vi "test Set and Get Options with GE Reflective Memory.vi"(8 "error in (no error)":errorcluster, 11 "TestCase in":refnum<class "Set and Get Config Options Test.lvclass">) -> (0 "error out":errorcluster, 3 "TestCase out":refnum<class "Set and Get Config Options Test.lvclass">)   [LabVIEW 2017, in "Set and Get Config Options Test.lvclass"]
uses:
  Set and Get Config Options Test.lvclass
  NationalInstruments.VeriStand.SystemDefinitionAPI
  <vilib>/addons/_JKI Toolkits/VI Tester/TestCase.llb/TestCase.lvclass
  niveristand-custom-device-testing-tools/VeriStandTestUtilities/VeriStandTestUtilities.lvlib
  C:/Program Files (x86)/National Instruments/LabVIEW 2017/vi.lib/addons/_JKI Toolkits/VI Tester/TestCase.llb/TestCase.lvclass
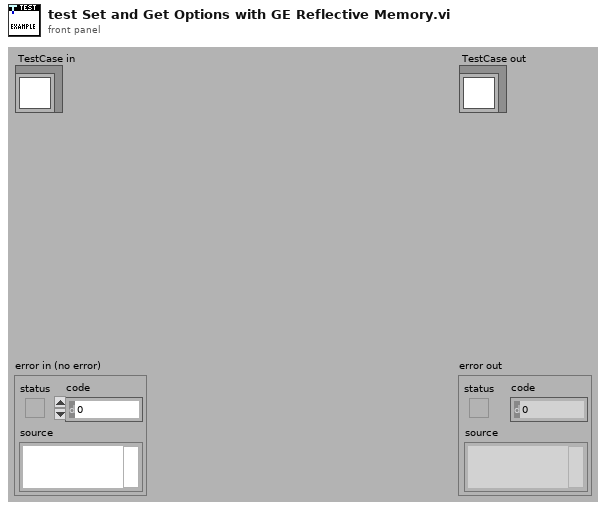
[diagram p1: front panel]
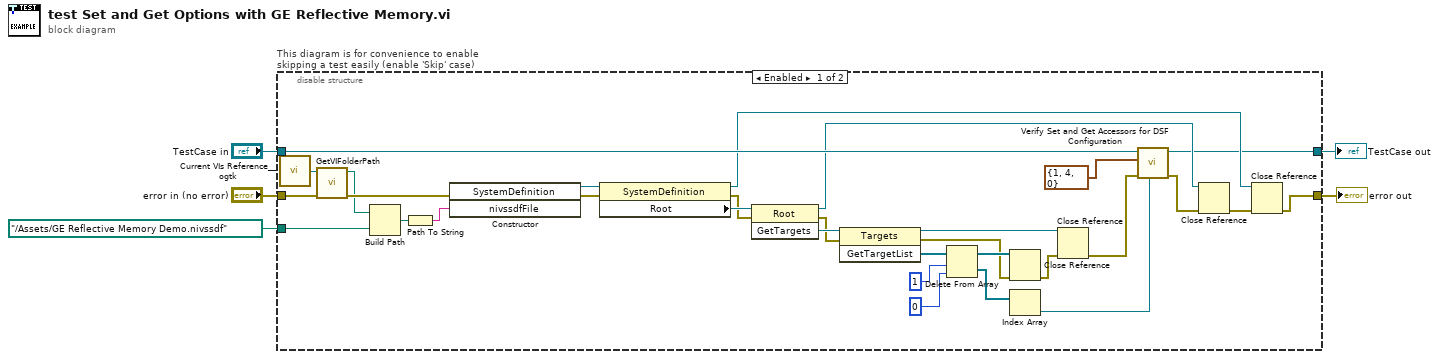
[diagram p0: block diagram]
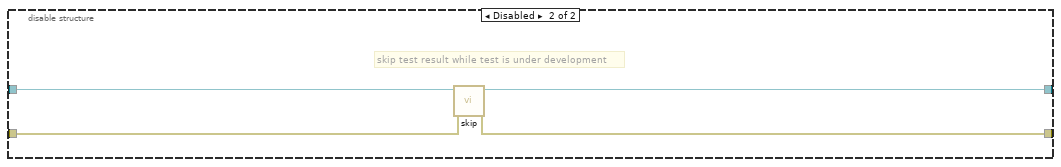
[diagram p2: hidden frame]
diagram:
  n1 = disable-structure "This diagram is for convenience to enable skipping a test easily (enable 'Skip' case)" shown="Enabled" {
    disable-tunnel: "TestCase in" -> [w36 w40]
    disable-tunnel: [w8 w38] -> w2
    disable-tunnel: [w10 w39] -> w4
    disable-tunnel: "error in (no error)" -> [w16 w37]
    disable-tunnel: path "../Assets/GE Reflective Memory Demo.nivssdf" ("Absolute or Relative Path") -> [w17 _]
    frame Enabled {
      n2 = call <userlib>:"Current VIs Reference__ogtk.vi"() -> ("Current VI's reference"=w19:refnum<vi>)  [unwired: 5 in]
      n3 = call "GetVIFolderPath.vi"("error in (no error)"=w16, "VI Reference in"=w19) -> ("error out"=w22:errorcluster, "VI Folder Path out"=w20:path)  [unwired: 8 in]
      n4 = Build Path(base path=w20, name or relative path=w17) -> (appended path=w21:path)
      n5 = Path To String(path=w21) -> (string=w24:string)
      n6 = constructor class="SystemDefinition" ("Constructor Node")(error in=w22, "nivssdfFile"=w24) -> (reference out=w25:refnum<k24>, error out=w23:errorcluster)  [unwired: 2 in, 2 out]
      n7 = property on="Property Node" class="SystemDefinition"(reference=w25, error in=w23) -> (reference out=w13:refnum<k24>, error out=w26:errorcluster, "Root"=w27:refnum<k24>)
      n8 = invoke on="Invoke Node" class="Root" method="GetTargets"(reference=w27, error in=w26) -> (reference out=w14:refnum<k24>, error out=w28:errorcluster, "GetTargets"=w29:refnum<k24>)  [unwired: 1 in]
      n9 = invoke on="Invoke Node" class="Targets" method="GetTargetList"(reference=w29, error in=w28) -> (reference out=w34:refnum<k24>, error out=w31:errorcluster, "GetTargetList"=w30:refnum<k24>[])  [unwired: 1 in]
      n10 = Delete From Array(array=w30, length=1, index=0) -> (deleted portion=w35:refnum<k24>[], array with subset deleted=w32:refnum<k24>[])
      n11 = Close Reference(reference=w32, error in (no error)=w31) -> (error out=w33:errorcluster)
      n12 = Index Array(array=w35) -> (element=w7:refnum<k24>)  [unwired: 1 in]
      n13 = Close Reference(reference=w34, error in (no error)=w33) -> (error out=w15:errorcluster)
      n14 = call "Verify Set and Get Accessors for DSF Configuration.vi"(".NET Refnum"=w7, "error in"=w15, "version"=cluster{"major":u32, "minor":u32, "update":u32} {"major"=1, "minor"=4, "update"=0}, "Set and Get Config Options Test in"=w36) -> ("error out"=w9:errorcluster, "Set and Get Config Options Test out"=w8:refnum<class "Set and Get Config Options Test.lvclass">)  [unwired: 6 in]
      n15 = Close Reference(reference=w14, error in (no error)=w9) -> (error out=w12:errorcluster)
      n16 = Close Reference(reference=w13, error in (no error)=w12) -> (error out=w10:errorcluster)
    }
    frame Disabled {
      # "skip test result while test is under development"
      n17 = call <vilib>:"skip.vi"("error in (no error)"=w37, "TestCase in"=w40) -> ("error out"=w39:errorcluster, "TestCase out"=w38:refnum<class "Set and Get Config Options Test.lvclass">)  [unwired: 8 in]
    }
  }
  "error out" <- w4
  "TestCase out" <- w2
